vi "ELVIS III v1.0 Shutdown Encoder.vi"(8 "error in (no error)":errorcluster, 10 "Channel":T1, 11 "myRIO Ref In":T2) -> (0 "error out":errorcluster, 3 "myRIO Ref Out":T2)   [LabVIEW 2021]
uses:
  <vilib>/myRIO/Common/Instrument Driver Framework/Utilities/typedefs/myRIO v1.0 Reference.ctl
  <vilib>/myRIO/Common/Instrument Driver Framework/Utilities/typedefs/Generic FPGA Reference.ctl
  <vilib>/myRIO/Common/Instrument Driver Framework/myRIO v1.0/Encoder/typedefs/Encoder Channels Enum.ctl
  <vilib>/myRIO/Common/Instrument Driver Framework/myRIO v1.0/Encoder/typedefs/Encoder Config Manager Action Enum.ctl
  <vilib>/myRIO/Common/Instrument Driver Framework/ELVIS III v1.0/Encoder/typedefs/ELVIS III Encoder Channels FPGA Reference.ctl
  <vilib>/rvi/errors/niLvFpgaAdjustHostInterfaceError.vi
  <vilib>/rvi/interface/nirviReadWriteControl/nirviReadWriteControl.xnode
  NiFpgaLv.dll
  <vilib>/rvi/interface/Simulation/niFpgaSimulationCallBeginRW.vi
panel:
  # "This VI turns off the specified Encoder channel and zeroes out all of its registers."
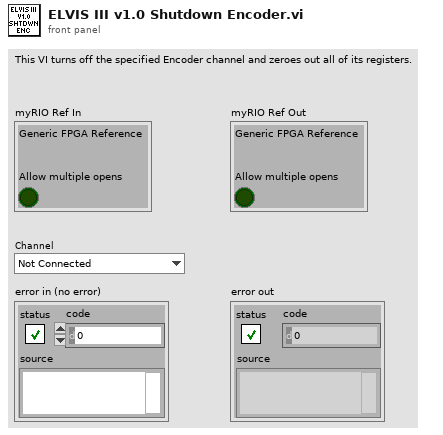
[diagram p1: front panel]
types:
  T1 = typedef "Encoder Channels Enum.ctl" = enum16{"Not Connected", "C/ENC0", "C/ENC1", "A/ENC", "A/ENC0", "A/ENC1", "A/ENC2", "A/ENC3", "A/ENC4", "A/ENC5", "A/ENC6", "A/ENC7", "A/ENC8", "A/ENC9", "B/ENC", "B/ENC0", "B/ENC1", "B/ENC2", "B/ENC3", "B/ENC4", "B/ENC5", "B/ENC6", "B/ENC7", "B/ENC8", "B/ENC9", "DIO/ENC0", "DIO/ENC1", "DIO/ENC2", "DIO/ENC3", "DIO/ENC4"}
  T2 = typedef "myRIO v1.0 Reference.ctl" = cluster{"Generic FPGA Reference":T3, "Allow multiple opens":bool}
  T3 = typedef "Generic FPGA Reference.ctl" = refnum<k20>
  T4 = typedef "Encoder Config Manager Action Enum.ctl" = enum16{"Do Nothing", "Store", "Clear"}
  T5 = typedef "ELVIS III Encoder Channels FPGA Reference.ctl" = refnum<k20>
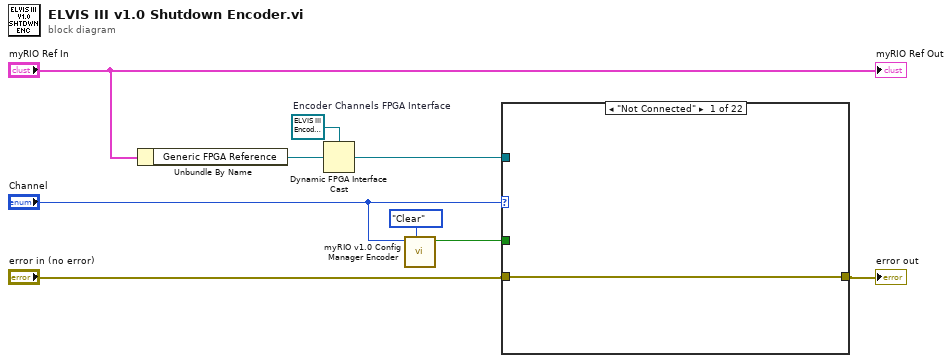
[diagram p0: block diagram]
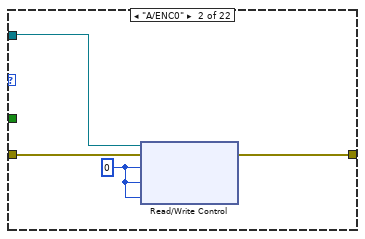
[diagram p2: hidden frame]
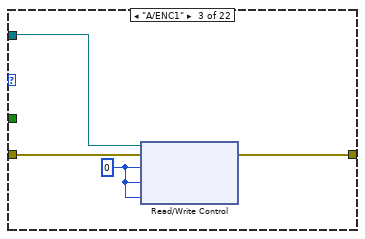
[diagram p3: hidden frame]
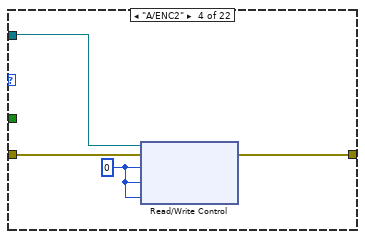
[diagram p4: hidden frame]
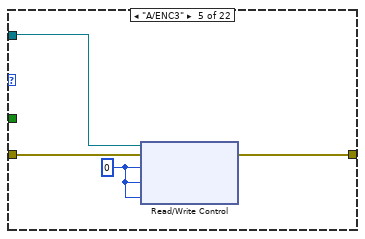
[diagram p5: hidden frame]
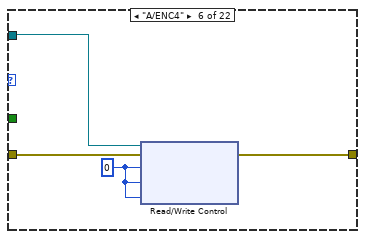
[diagram p6: hidden frame]
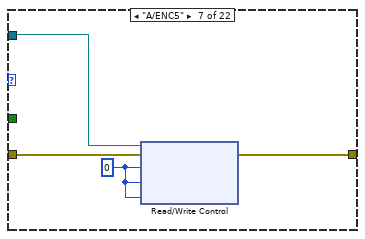
[diagram p7: hidden frame]
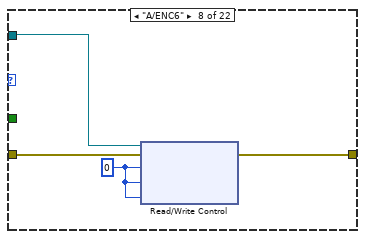
[diagram p8: hidden frame]
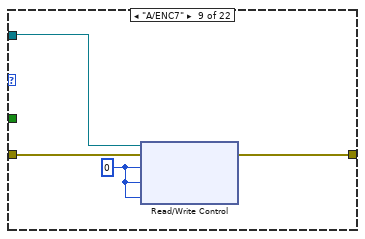
[diagram p9: hidden frame]
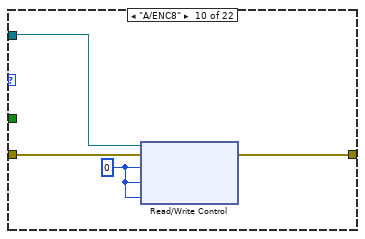
[diagram p10: hidden frame]
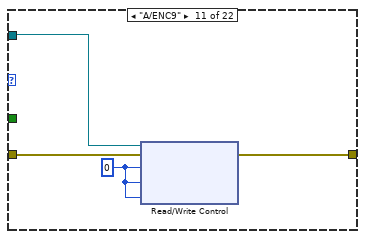
[diagram p11: hidden frame]
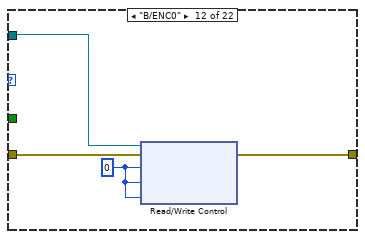
[diagram p12: hidden frame]
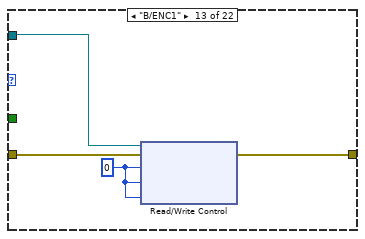
[diagram p13: hidden frame]
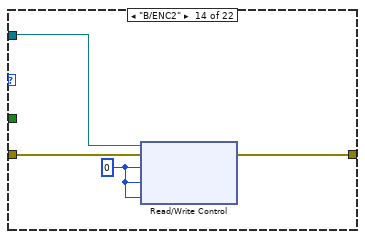
[diagram p14: hidden frame]
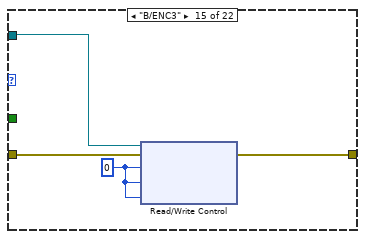
[diagram p15: hidden frame]
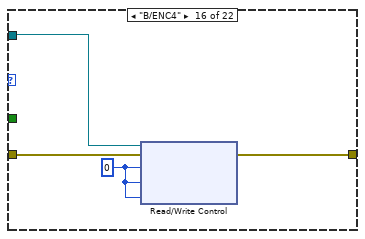
[diagram p16: hidden frame]
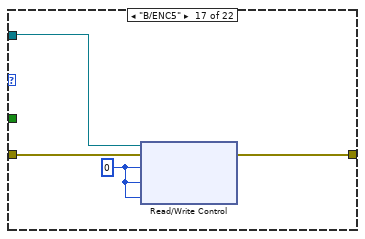
[diagram p17: hidden frame]
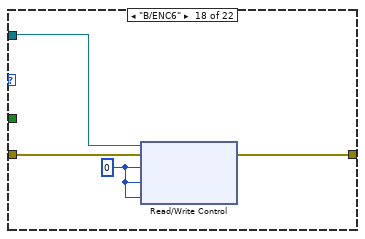
[diagram p18: hidden frame]
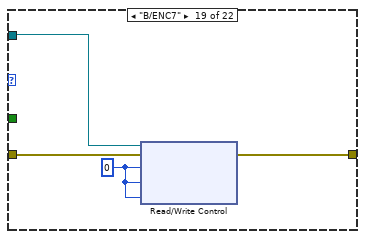
[diagram p19: hidden frame]
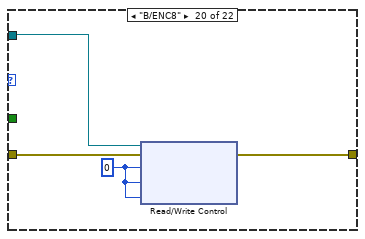
[diagram p20: hidden frame]
diagram:
  w9 = T5 refnum  # Encoder Channels FPGA Interface
  n1 = Unbundle By Name("myRIO Ref In") -> ("Generic FPGA Reference"=w8:T3)
  n2 = Dynamic FPGA Interface Cast(Session In=w9, Type=w8) -> (Session Out=w1:T5)
  n3 = call <vilib>:"myRIO v1.0 Config Manager Encoder.vi"("Action"=Encoder_Config_Manager_Action_Enum."Clear", "Encoder Channel"="Channel") -> ("Success?"=w3:bool)  [unwired: 9 in]
  n4 = case shown="\"Not Connected\"" "Channel" {
    tunnel: "error in (no error)" -> [w10 w12 w16 w20 w24 w28 w32 w36 w40 w44 w48 w52 w56 w60 w64 w68 w72 w76 w80 w84 w88 w91]
    tunnel: [w10 w11 w15 w19 w23 w27 w31 w35 w39 w43 w47 w51 w55 w59 w63 w67 w71 w75 w79 w83 w87 w92] -> w4
    tunnel: w3 -> [_ _ _ _ _ _ _ _ _ _ _ _ _ _ _ _ _ _ _ _ _ _]
    tunnel: w1 -> [_ w13 w17 w21 w25 w29 w33 w37 w41 w45 w49 w53 w57 w61 w65 w69 w73 w77 w81 w85 w89 _]
    frame "Not Connected" {
    }
    frame "A/ENC0" {
      w14 = u8 0 ("ENC.C_0.CNFG")
      n5 = xnode "Read/Write Control"("FPGA VI Reference In"=w13, "error in"=w12, "ENC.A_0.CNFG"=w14, "ENC.A_0.CNTR"=w14, "ENC.A_0.STAT"=w14) -> ("error out"=w11:errorcluster)  [unwired: 1 out]
    }
    frame "A/ENC1" {
      w18 = u8 0 ("ENC.C_0.CNFG")
      n6 = xnode "Read/Write Control"("FPGA VI Reference In"=w17, "error in"=w16, "ENC.A_1.CNFG"=w18, "ENC.A_1.CNTR"=w18, "ENC.A_1.STAT"=w18) -> ("error out"=w15:errorcluster)  [unwired: 1 out]
    }
    frame "A/ENC2" {
      w22 = u8 0 ("ENC.C_0.CNFG")
      n7 = xnode "Read/Write Control"("FPGA VI Reference In"=w21, "error in"=w20, "ENC.A_2.CNFG"=w22, "ENC.A_2.CNTR"=w22, "ENC.A_2.STAT"=w22) -> ("error out"=w19:errorcluster)  [unwired: 1 out]
    }
    frame "A/ENC3" {
      w26 = u8 0 ("ENC.C_0.CNFG")
      n8 = xnode "Read/Write Control"("FPGA VI Reference In"=w25, "error in"=w24, "ENC.A_3.CNFG"=w26, "ENC.A_3.CNTR"=w26, "ENC.A_3.STAT"=w26) -> ("error out"=w23:errorcluster)  [unwired: 1 out]
    }
    frame "A/ENC4" {
      w30 = u8 0 ("ENC.C_0.CNFG")
      n9 = xnode "Read/Write Control"("FPGA VI Reference In"=w29, "error in"=w28, "ENC.A_4.CNFG"=w30, "ENC.A_4.CNTR"=w30, "ENC.A_4.STAT"=w30) -> ("error out"=w27:errorcluster)  [unwired: 1 out]
    }
    frame "A/ENC5" {
      w34 = u8 0 ("ENC.C_0.CNFG")
      n10 = xnode "Read/Write Control"("FPGA VI Reference In"=w33, "error in"=w32, "ENC.A_5.CNFG"=w34, "ENC.A_5.CNTR"=w34, "ENC.A_5.STAT"=w34) -> ("error out"=w31:errorcluster)  [unwired: 1 out]
    }
    frame "A/ENC6" {
      w38 = u8 0 ("ENC.C_0.CNFG")
      n11 = xnode "Read/Write Control"("FPGA VI Reference In"=w37, "error in"=w36, "ENC.A_6.CNFG"=w38, "ENC.A_6.CNTR"=w38, "ENC.A_6.STAT"=w38) -> ("error out"=w35:errorcluster)  [unwired: 1 out]
    }
    frame "A/ENC7" {
      w42 = u8 0 ("ENC.C_0.CNFG")
      n12 = xnode "Read/Write Control"("FPGA VI Reference In"=w41, "error in"=w40, "ENC.A_7.CNFG"=w42, "ENC.A_7.CNTR"=w42, "ENC.A_7.STAT"=w42) -> ("error out"=w39:errorcluster)  [unwired: 1 out]
    }
    frame "A/ENC8" {
      w46 = u8 0 ("ENC.C_0.CNFG")
      n13 = xnode "Read/Write Control"("FPGA VI Reference In"=w45, "error in"=w44, "ENC.A_8.CNFG"=w46, "ENC.A_8.CNTR"=w46, "ENC.A_8.STAT"=w46) -> ("error out"=w43:errorcluster)  [unwired: 1 out]
    }
    frame "A/ENC9" {
      w50 = u8 0 ("ENC.C_0.CNFG")
      n14 = xnode "Read/Write Control"("FPGA VI Reference In"=w49, "error in"=w48, "ENC.A_9.CNFG"=w50, "ENC.A_9.CNTR"=w50, "ENC.A_9.STAT"=w50) -> ("error out"=w47:errorcluster)  [unwired: 1 out]
    }
    frame "B/ENC0" {
      w54 = u8 0 ("ENC.C_0.CNFG")
      n15 = xnode "Read/Write Control"("FPGA VI Reference In"=w53, "error in"=w52, "ENC.B_0.CNFG"=w54, "ENC.B_0.CNTR"=w54, "ENC.B_0.STAT"=w54) -> ("error out"=w51:errorcluster)  [unwired: 1 out]
    }
    frame "B/ENC1" {
      w58 = u8 0 ("ENC.C_0.CNFG")
      n16 = xnode "Read/Write Control"("FPGA VI Reference In"=w57, "error in"=w56, "ENC.B_1.CNFG"=w58, "ENC.B_1.CNTR"=w58, "ENC.B_1.STAT"=w58) -> ("error out"=w55:errorcluster)  [unwired: 1 out]
    }
    frame "B/ENC2" {
      w62 = u8 0 ("ENC.C_0.CNFG")
      n17 = xnode "Read/Write Control"("FPGA VI Reference In"=w61, "error in"=w60, "ENC.B_2.CNFG"=w62, "ENC.B_2.CNTR"=w62, "ENC.B_2.STAT"=w62) -> ("error out"=w59:errorcluster)  [unwired: 1 out]
    }
    frame "B/ENC3" {
      w66 = u8 0 ("ENC.C_0.CNFG")
      n18 = xnode "Read/Write Control"("FPGA VI Reference In"=w65, "error in"=w64, "ENC.B_3.CNFG"=w66, "ENC.B_3.CNTR"=w66, "ENC.B_3.STAT"=w66) -> ("error out"=w63:errorcluster)  [unwired: 1 out]
    }
    frame "B/ENC4" {
      w70 = u8 0 ("ENC.C_0.CNFG")
      n19 = xnode "Read/Write Control"("FPGA VI Reference In"=w69, "error in"=w68, "ENC.B_4.CNFG"=w70, "ENC.B_4.CNTR"=w70, "ENC.B_4.STAT"=w70) -> ("error out"=w67:errorcluster)  [unwired: 1 out]
    }
    frame "B/ENC5" {
      w74 = u8 0 ("ENC.C_0.CNFG")
      n20 = xnode "Read/Write Control"("FPGA VI Reference In"=w73, "error in"=w72, "ENC.B_5.CNFG"=w74, "ENC.B_5.CNTR"=w74, "ENC.B_5.STAT"=w74) -> ("error out"=w71:errorcluster)  [unwired: 1 out]
    }
    frame "B/ENC6" {
      w78 = u8 0 ("ENC.C_0.CNFG")
      n21 = xnode "Read/Write Control"("FPGA VI Reference In"=w77, "error in"=w76, "ENC.B_6.CNFG"=w78, "ENC.B_6.CNTR"=w78, "ENC.B_6.STAT"=w78) -> ("error out"=w75:errorcluster)  [unwired: 1 out]
    }
    frame "B/ENC7" {
      w82 = u8 0 ("ENC.C_0.CNFG")
      n22 = xnode "Read/Write Control"("FPGA VI Reference In"=w81, "error in"=w80, "ENC.B_7.CNFG"=w82, "ENC.B_7.CNTR"=w82, "ENC.B_7.STAT"=w82) -> ("error out"=w79:errorcluster)  [unwired: 1 out]
    }
    frame "B/ENC8" {
      w86 = u8 0 ("ENC.C_0.CNFG")
      n23 = xnode "Read/Write Control"("FPGA VI Reference In"=w85, "error in"=w84, "ENC.B_8.CNFG"=w86, "ENC.B_8.CNTR"=w86, "ENC.B_8.STAT"=w86) -> ("error out"=w83:errorcluster)  [unwired: 1 out]
    }
    frame "B/ENC9" {
      w90 = u8 0 ("ENC.C_0.CNFG")
      n24 = xnode "Read/Write Control"("FPGA VI Reference In"=w89, "error in"=w88, "ENC.B_9.CNFG"=w90, "ENC.B_9.CNTR"=w90, "ENC.B_9.STAT"=w90) -> ("error out"=w87:errorcluster)  [unwired: 1 out]
    }
    frame Default {
      # "The channel requested is not supported. This happens when the channel name is valid (a valid channel enum) but there it is not handled in the case structure."
      n25 = call <vilib>:"Error Cluster From Error Code.vi"("error in (no error)"=w91, "error code (0)"=-363003) -> ("error out"=w92:errorcluster)  [unwired: 7 in]
    }
  }
  "error out" <- w4
  "myRIO Ref Out" <- "myRIO Ref In"
